vi "Test Waveform log.vi"() -> ()   [LabVIEW 2016]
uses:
  <vilib>/xnet/xnet.llb/XNET Read (Signal Waveform) .vi
panel:
  in  "stop":bool
  out "Waveform Chart":waveform(dbl)[](graph)
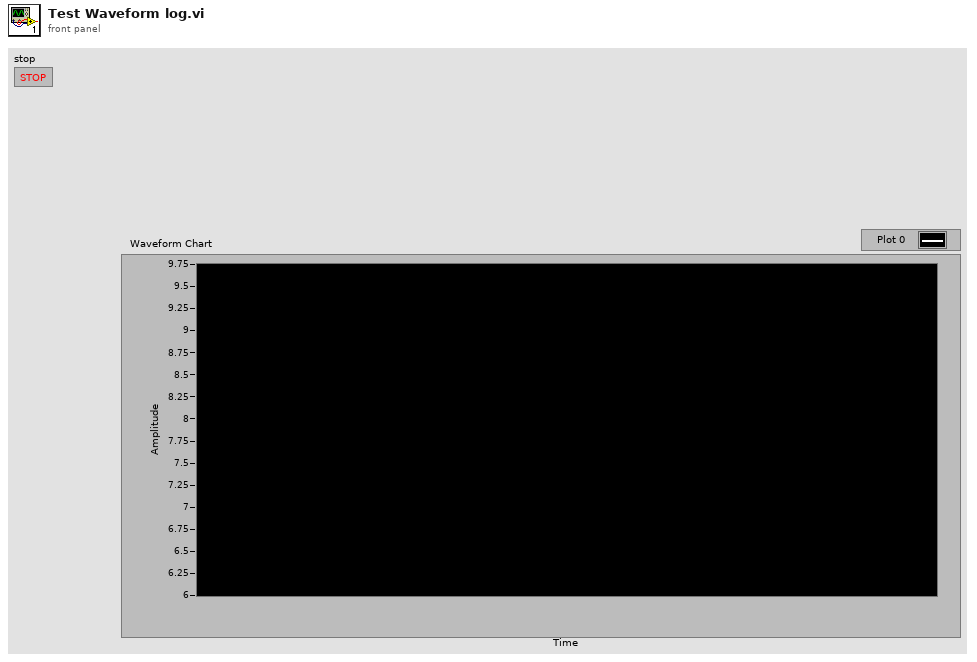
[diagram p1: front panel]
types:
  T1 = enum16{"open", "open or create", "create or replace", "create", "open (read-only)"}
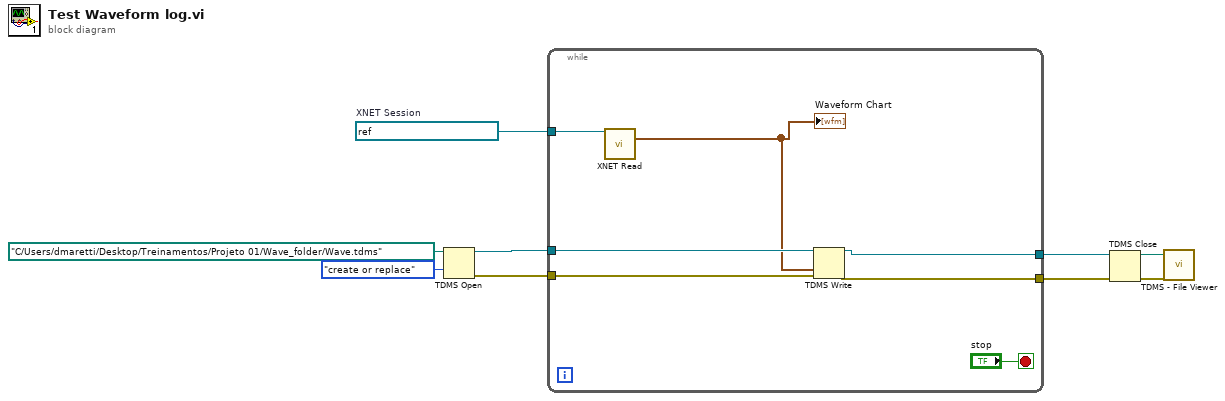
[diagram p0: block diagram]
diagram:
  w9 = refnum<k21> "New NI-XNET Session"  # XNET Session
  n1 = TDMS Open(10:T1."create or replace" ("operation (0:open)"), 11:path "C:/Users/dmaretti/Desktop/Treinamentos/Projeto 01/Wave_folder/Wave.tdms" ("file path")) -> (0:w3:errorcluster, 3:w6:refnum<k34>)  [unwired: 5 in]
  n2 = while {
    tunnel: w9 -> [w16]
    tunnel: w6 -> [w15]
    tunnel: [w14] -> w5
    tunnel: [w13] -> w4
    tunnel: w3 -> [w12]
    stop <- "stop" stop-if-true
    n3 = call-poly <vilib>:"XNET Read.vi"("session in"=w16) -> ("data"=w11:waveform(dbl)[])  [unwired: 12 in, 2 out]
    "Waveform Chart" <- w11
    n4 = TDMS Write(0:w15, 9:w11, 11:w12) -> (4:w14:refnum<k34>, 15:w13:errorcluster)  [unwired: 3 in, 2 out]
  }
  n5 = TDMS Close(8:w4, 11:w5) -> (0:w8:errorcluster, 3:w7:path)
  n6 = call <vilib>:"TDMS - File Viewer.vi"("error in (no error)"=w8, "file path"=w7) -> ()  [unwired: 4 in, 2 out]
